vi "Test 1 Race 3.vi"(8 "error in (no error)":errorcluster, 11 "Test Case In":refnum<class "Day 6 Test.lvclass">) -> (0 "error out":errorcluster, 3 "Test Case Out":refnum<class "Day 6 Test.lvclass">)   [LabVIEW 2021, in "Day 6 Test.lvclass"]
uses:
  Day 6 Test.lvclass
  C:/Program Files (x86)/National Instruments/LabVIEW 2021/vi.lib/Astemes/LUnit/Test Case.lvclass
  <vilib>/Astemes/LUnit/Test Case.lvclass/Test Case.ctl
  4993e8ee-a06a-463a-9684-69129f64d5ce.vi
  <vilib>/Astemes/LUnit/Append Pass Result.vi
  <vilib>/Astemes/LUnit/Append Fail Result.vi
  <vilib>/Astemes/LUnit/Describe Comparison.vi
  <vilib>/Astemes/LUnit/Compare Variants.vi
  <vilib>/Astemes/LUnit/Variant to string.vi
  <vilib>/Utility/Data Type/Get Type Information.vi
  <vilib>/Utility/LVClass/Get LV Class Name.vi
  Day 6 Test.lvclass/Day 6 Test.ctl
  Race/Race.lvclass
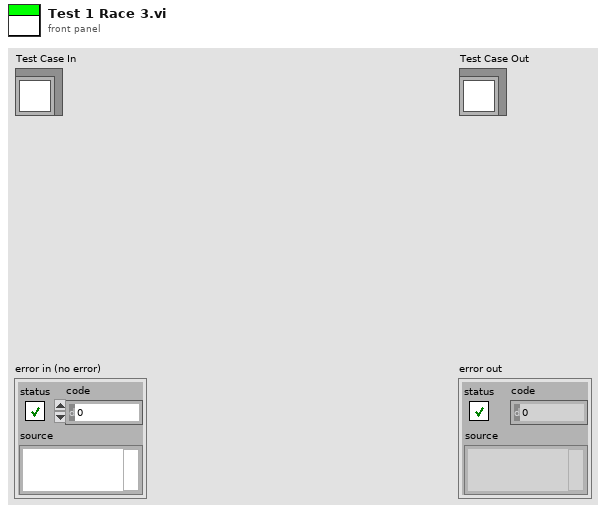
[diagram p1: front panel]
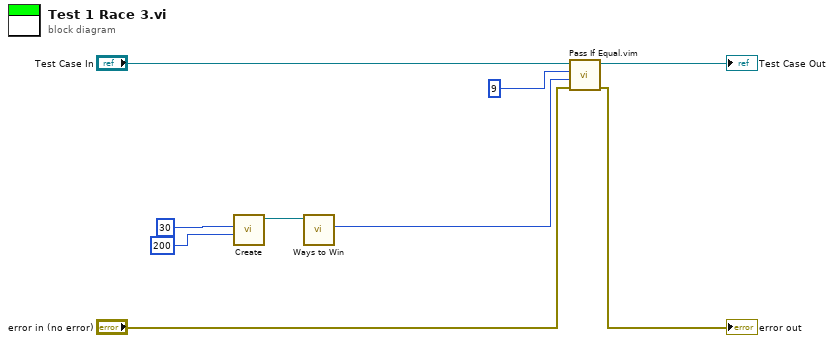
[diagram p0: block diagram]
diagram:
  n1 = call "Create.vi"("Distance"=u32 200, "Time"=u32 30) -> ("Race Out"=w3:refnum<class "Race.lvclass">)  [unwired: 8 in, 1 out]
  n2 = call "Ways to Win.vi"("Race In"=w3) -> ("Ways to win"=w2:u64)  [unwired: 9 in, 1 out]
  n3 = call "Pass If Equal.vim"("error in (no error)"="error in (no error)", "Actual"=w2, "Expected"=u32 9 ("Ways to win"), "LUnit Test Case In"="Test Case In") -> ("error out"=→"error out":errorcluster, "LUnit Test Case Out"=→"Test Case Out":refnum<class "Day 6 Test.lvclass">)  [unwired: 6 in]
